vi "ARD-LTC2499_EEPROM.vi"   [LabVIEW 2014]
uses:
  QwaveSys_Interface/QwaveSys_Interface.lvlib
  QwaveSys_ESP8266/QwaveSys_ESP8266.lvlib
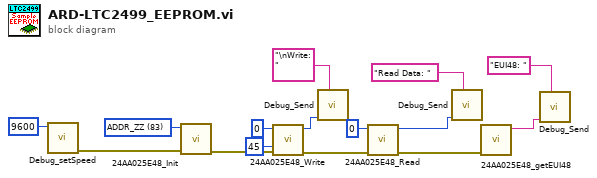
[diagram p0: block diagram]
diagram:
  w15 = u8 83 items=["ADDR_00"=80, "ADDR_0Z"=81, "ADDR_Z0"=82, "ADDR_ZZ"=83] ("Address")
  n1 = call "Debug_setSpeed.vi"("Speed"=u32 9600) -> ("error out"=w10:errorcluster)  [unwired: 10 in]
  n2 = call "24AA025E48_Init.vi"("error in (no error)"=w10, "Address"=w15) -> ("error out"=w14:errorcluster)  [unwired: 9 in]
  n3 = call "24AA025E48_Write.vi"("error in (no error)"=w14, "Data"=u8 45, "Address"=u16 0) -> ("error out"=w13:errorcluster, "error"=w7:u8)  [unwired: 7 in]
  n4 = call "Debug_Send.vi"("Name"="\nWrite: ", "DATA"=w7) -> ()  [unwired: 10 in]
  n5 = call "24AA025E48_Read.vi"("error in (no error)"=w13, "Address"=u16 0) -> ("error out"=w3:errorcluster, "Data"=w4:u8)  [unwired: 8 in]
  n6 = call "Debug_Send.vi"("Name"="Read Data: ", "DATA"=w4) -> ()  [unwired: 10 in]
  n7 = call "24AA025E48_getEUI48.vi"("error in (no error)"=w3) -> ("EUI48"=w2:string)  [unwired: 9 in, 1 out]
  n8 = call "Debug_Send.vi"("Name"="EUI48: ", "DATA"=w2) -> ()  [unwired: 10 in]
